vi "GetJSONData.vi"(0 "reference in":refnum<class "Graph.lvclass">, 2 "VI Reference":refnum<vi>, 5 "error in (no error)":errorcluster) -> (14 "reference out":refnum<class "Graph.lvclass">, 15 "JSON string":string, 19 "error out":errorcluster)   [LabVIEW 2014, in "Graph.lvclass"]
uses:
  Graph.lvclass
  <vilib>/Analysis/1siggen.llb/Ramp Pattern by Samples.vi
  <userlib>/_OpenG.lib/array/array.llb/Remove Duplicates from 1D Array (U32)__ogtk.vi
  <userlib>/_OpenG.lib/array/array.llb/Delete Elements from 1D Array (String)__ogtk.vi
  Object_class/Object.lvclass
  <vilib>/gmath/NI_Gmath.lvlib
  <vilib>/Analysis/NI_AALBase.lvlib
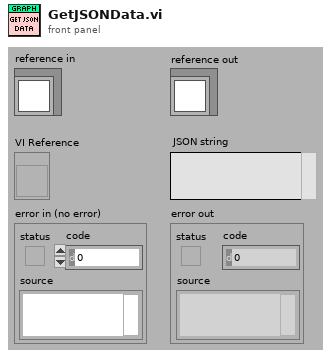
[diagram p1: front panel]
types:
  T1 = typedef "Object.lvclass/Attributes.ctl" = cluster{"UID":i32, "Type":string, "Coordinates":T2, "Reference":refnum<vi>}
  T2 = typedef "Object.lvclass/Coordinates.ctl" = cluster{"Left":i32, "Top":i32, "Height":u32, "Width":u32}
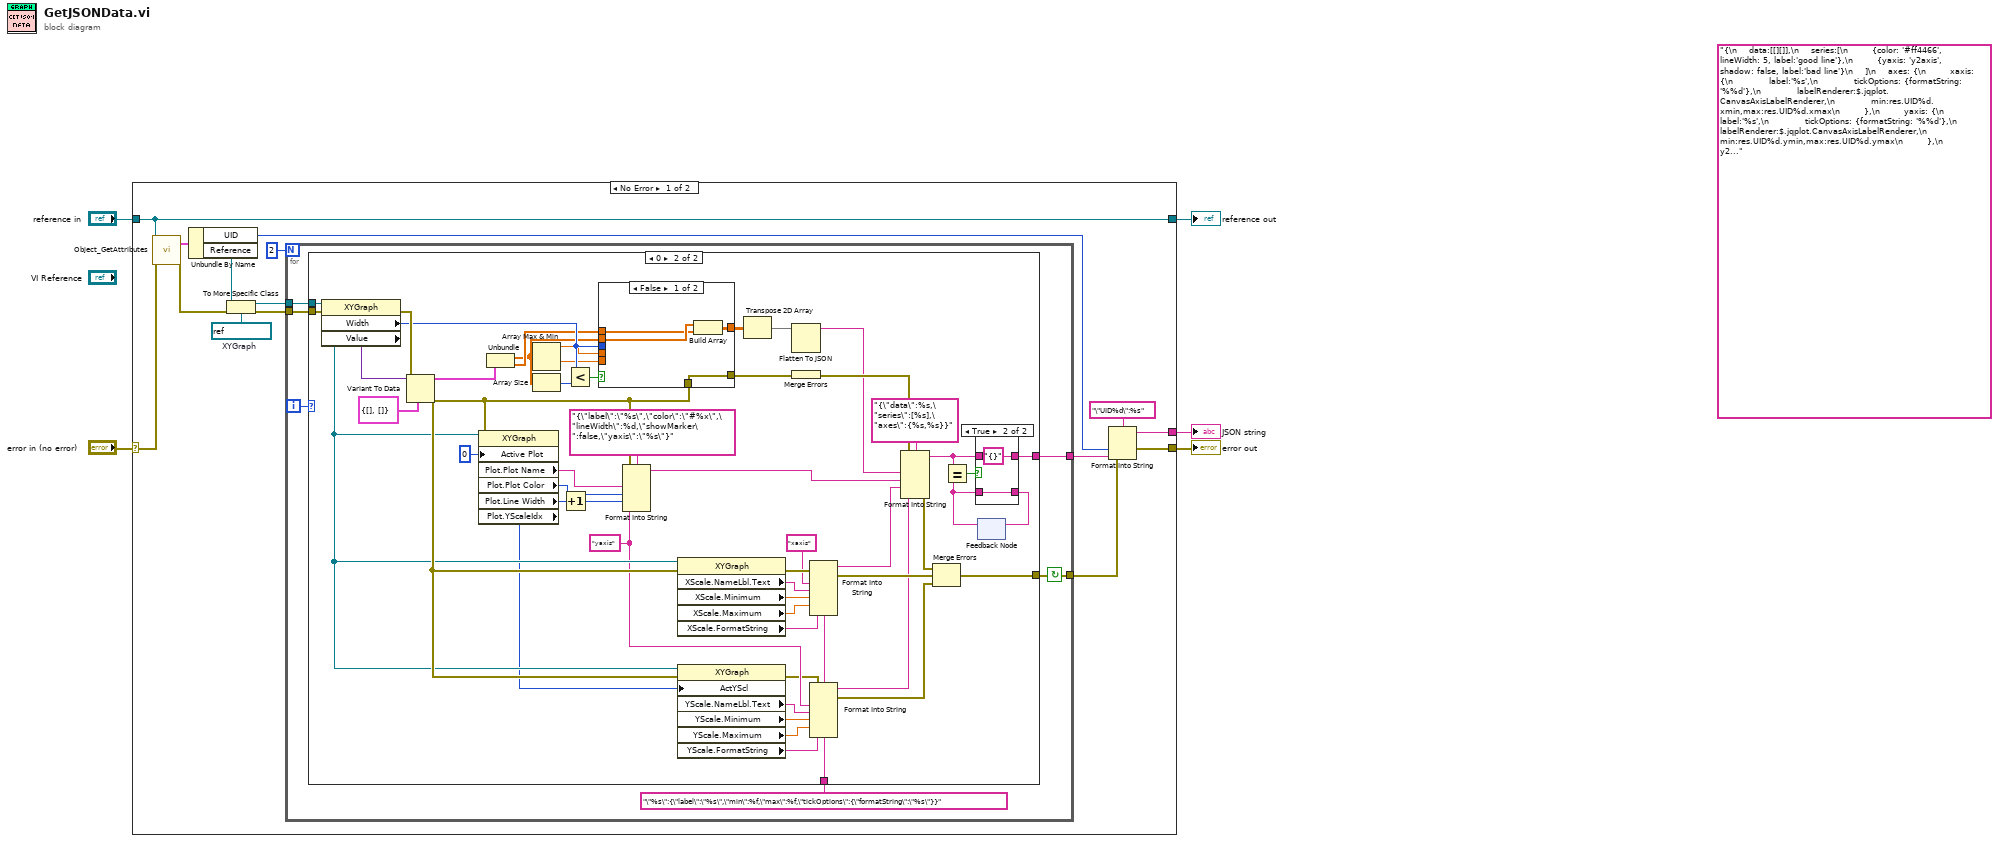
[diagram p0: block diagram]
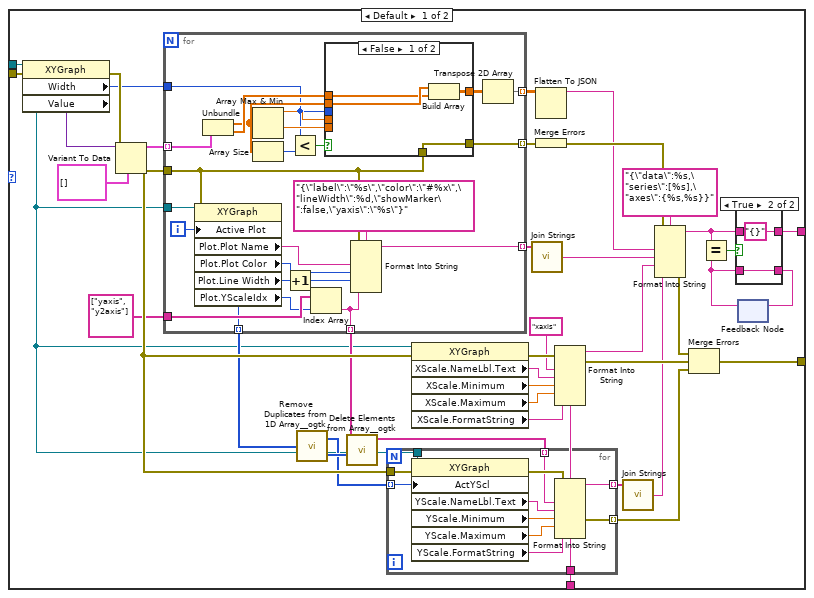
[diagram p2: hidden frame]
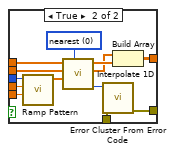
[diagram p4: hidden frame]
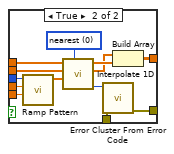
[diagram p5: hidden frame]
diagram:
  (unwired) "{\n    data:[[][]],\n    series:[\n        {color: '#ff4466', lineWidth: 5, label:'good line'},\n        {yaxis: 'y2axis', shadow: false, label:'bad line'}\n    ]\n    axes: {\n        xaxis: {\n            label:'%s',\n            tickOptions: {formatString: '%%d'},\n            labelRenderer:$.jqplot.CanvasAxisLabelRenderer,\n            min:res.UID%d.xmin,max:res.UID%d.xmax\n        },\n        yaxis: {\n            label:'%s',\n            tickOptions: {formatString: '%%d'},\n            labelRenderer:$.jqplot.CanvasAxisLabelRenderer,\n            min:res.UID%d.ymin,max:res.UID%d.ymax\n        },\n        y2axis: {\n            label:'%s',\n            tickOptions: {formatString: '%%d'},\n            labelRenderer:$.jqplot.CanvasAxisLabelRenderer\n        }\n      resetAxes:true\n    }\n}"
  n1 = case shown="No Error" "error in (no error)" {
    selector: "error in (no error)" -> [w18 w195]
    tunnel: [w19 w195] -> w4
    tunnel: [w11 w194] -> w2
    tunnel: "reference in" -> [w11 w194]
    tunnel: [w8 _] -> w1
    frame No Error {
      w12 = refnum<vi> refnum  # XYGraph
      n2 = call "Object_GetAttributes.vi"("reference in"=w11, "error in (no error)"=w18) -> ("Data"=w14:T1, "error out"=w16:errorcluster)  [unwired: 14 in, 2 out]
      n3 = Unbundle By Name(w14) -> ("UID"=w13:i32, "Reference"=w7:refnum<vi>)
      n4 = To More Specific Class(target class=w12, reference=w7, error in=w16) -> (specific class reference=w9:refnum<vi>, error out=w17:errorcluster)
      n5 = for {
        N: 2 -> [_]
        tunnel: [w25] -> w20
        tunnel: w17 -> [w26]
        tunnel: w9 -> [w23]
        tunnel: [w21] -> w6
        i -> [w24]
        stop <- w25 continue-if-true
        n6 = case shown="0" w24 {
          tunnel: w23 -> [w29 w147]
          tunnel: w26 -> [w60 w167]
          tunnel: [w59 w166] -> w25
          tunnel: "\"%s\":{\"label\":\"%s\",\"min\":%f,\"max\":%f,\"tickOptions\":{\"formatString\":\"%s\"}}" -> [w28 w146]
          tunnel: [w27 w145] -> w21
          frame Default {
            n7 = property class="XYGraph"(reference=w29, error in=w60) -> (error out=w66:errorcluster, "Width"=w34:u32, "Value"=w56:variant)  [unwired: 1 out]
            n8 = Variant To Data(error in=w66, type=cluster{dbl[], dbl[]}[] [], Variant=w56) -> (data=w54:cluster{dbl[], dbl[]}[], error out=w65:errorcluster)
            n9 = for {
              tunnel: [w102] -> w36 mode=indexing
              tunnel: w54 -> [w99] mode=indexing
              tunnel: w29 -> [w86]
              tunnel: [w104] -> w58 mode=indexing
              tunnel: w34 -> [w93]
              tunnel: w65 -> [w103]
              tunnel: string[] ["yaxis", "y2axis"] -> [w87]
              tunnel: [w85] -> w39 mode=indexing
              tunnel: [w84] -> w38 mode=indexing
              tunnel: [w83] -> w37 mode=indexing
              i -> [w88]
              n10 = property on="Property Node" class="XYGraph"(reference=w86, error in=w103, "Active Plot"=w88) -> ("Plot.Plot Name"=w90:string, "Plot.Plot Color"=w91:u32, "Plot.Line Width"=w92:u8, "Plot.YScaleIdx"=w85:u32)  [unwired: 2 out]
              n11 = Unbundle(w99) -> (w95:dbl[], w100:dbl[])
              n12 = Array Max & Min(array=w95) -> (max value=w98:dbl, min value=w97:dbl)  [unwired: 2 out]
              n13 = Array Size(array=w95) -> (size(s)=w94:i32)
              n14 = Increment(x=w92) -> (x+1=w82:u8)
              n15 = Less?(x=w93, y=w94) -> (x < y?=w96:bool)
              n16 = Index Array(array=w87, index=w85) -> (element=w84:string)
              n17 = case shown="False" w96 {
                tunnel: [w108 w121] -> w104
                tunnel: [w107 w119] -> w101
                tunnel: w100 -> [w105 w118]
                tunnel: w95 -> [w106 w112]
                tunnel: w98 -> [_ w111]
                tunnel: w97 -> [_ w110]
                tunnel: w93 -> [_ w109]
                tunnel: w103 -> [w108 w120]
                frame False {
                  n18 = Build Array(w106, w105) -> (w107:dbl[][])
                }
                frame True {
                  w113 = 0 items=["nearest", "linear", "spline", "cubic Hermite", "Lagrange"] ("method")
                  n19 = call-poly <vilib>:"Ramp Pattern.vi"("start"=w110, "end"=w111, "samples"=w109) -> ("Ramp Pattern"=w114:dbl[])  [unwired: 7 in, 1 out]
                  n20 = call <vilib>:"Interpolate 1D.vi"("method"=w113, "xi"=w114, "X"=w112, "Y"=w118) -> ("error"=w115:i32, "xi used"=w116:dbl[], "yi"=w117:dbl[])  [unwired: 5 in]
                  n21 = call <vilib>:"Error Cluster From Error Code.vi"("error in (no error)"=w120, "error code (0)"=w115) -> ("error out"=w121:errorcluster)  [unwired: 7 in]
                  n22 = Build Array(w116, w117) -> (w119:dbl[][])
                }
              }
              n23 = Format Into String(format string="{\"label\":\"%s\",\"color\":\"#%x\",\"lineWidth\":%d,\"showMarker\":false,\"yaxis\":\"%s\"}", error in=w103, w90, w91, w82, w84) -> (resulting string=w83:string)  [unwired: 1 in, 1 out]
              n24 = Transpose 2D Array(2D array=w101) -> (transposed array=w102:dbl[][])
            }
            n25 = call-poly <userlib>:"Remove Duplicates from 1D Array__ogtk.vi"("Input Array"=w39) -> ("Output Array"=w40:u32[], "indices of removed elements"=w51:i32[])
            n26 = call-poly <userlib>:"Delete Elements from Array__ogtk.vi"("indices"=w51, "array"=w38) -> ("array w/ subset deleted"=w52:string[])  [unwired: 8 in, 1 out]
            n27 = for {
              tunnel: w40 -> [w78] mode=indexing
              tunnel: w52 -> [w76] mode=indexing
              tunnel: [w72] -> w41 mode=indexing
              tunnel: w28 -> [w71]
              tunnel: w29 -> [w70]
              tunnel: w65 -> [w81]
              tunnel: [w79] -> w57 mode=indexing
              n28 = property on="Property Node" class="XYGraph"(reference=w70, error in=w81, "ActYScl"=w78) -> (error out=w80:errorcluster, "YScale.NameLbl.Text"=w77:string, "YScale.Minimum"=w75:dbl, "YScale.Maximum"=w74:dbl, "YScale.FormatString"=w73:string)  [unwired: 1 out]
              n29 = Format Into String(format string=w71, error in=w80, w76, w77, w75, w74, w73) -> (resulting string=w72:string, error out=w79:errorcluster)  [unwired: 1 in]
            }
            n30 = property on="Property Node" class="XYGraph"(reference=w29, error in=w65) -> (error out=w64:errorcluster, "XScale.NameLbl.Text"=w45:string, "XScale.Minimum"=w46:dbl, "XScale.Maximum"=w47:dbl, "XScale.FormatString"=w48:string)  [unwired: 1 out]
            n31 = call <vilib>:"Join Strings.vi"("Strings In"=w37) -> ("String"=w44:string)  [unwired: 2 in]
            n32 = Flatten To JSON(anything=w36) -> (JSON string=w35:string)  [unwired: 2 in, 1 out]
            n33 = Merge Errors(w58) -> (w63:errorcluster)
            n34 = Format Into String(format string=w28, error in=w64, "xaxis", w45, w46, w47, w48) -> (resulting string=w49:string, error out=w62:errorcluster)  [unwired: 1 in]
            n35 = call <vilib>:"Join Strings.vi"("Strings In"=w41) -> ("String"=w43:string)  [unwired: 2 in]
            n36 = Format Into String(format string="{\"data\":%s,\"series\":[%s],\"axes\":{%s,%s}}", error in=w63, w35, w44, w49, w43) -> (resulting string=w30:string, error out=w61:errorcluster)  [unwired: 1 in]
            n37 = Merge Errors(w61, w62, w57) -> (w59:errorcluster)
            n38 = feedback #1() -> (w31:string)  [unwired: 1 in]
            n39 = Equal?(x=w30, y=w31) -> (x = y?=w33:bool)
            n40 = case shown="True" w33 {
              tunnel: [w67 w69] -> w32
              tunnel: w31 -> [_ w69]
              tunnel: w30 -> [w67 _]
              tunnel: [w67 "{}"] -> w27
              frame False {
              }
              frame True {
              }
            }
            n41 = feedback-in #1(w32) -> ()
          }
          frame 0 {
            w129 = "yaxis"
            n42 = property class="XYGraph"(reference=w147, error in=w167) -> (error out=w173:errorcluster, "Width"=w152:u32, "Value"=w163:variant)  [unwired: 1 out]
            n43 = Variant To Data(error in=w173, type=cluster{dbl[], dbl[]} {[], []}, Variant=w163) -> (data=w162:cluster{dbl[], dbl[]}, error out=w172:errorcluster)
            n44 = property on="Property Node" class="XYGraph"(reference=w147, error in=w172, "Active Plot"=u32 0) -> ("Plot.Plot Name"=w134:string, "Plot.Plot Color"=w135:u32, "Plot.Line Width"=w136:u8, "Plot.YScaleIdx"=w128:u32)  [unwired: 2 out]
            n45 = Unbundle(w162) -> (w138:dbl[], w142:dbl[])
            n46 = Array Max & Min(array=w138) -> (max value=w141:dbl, min value=w140:dbl)  [unwired: 2 out]
            n47 = Array Size(array=w138) -> (size(s)=w137:i32)
            n48 = Increment(x=w136) -> (x+1=w132:u8)
            n49 = Less?(x=w152, y=w137) -> (x < y?=w139:bool)
            n50 = case shown="False" w139 {
              tunnel: [w177 w190] -> w165
              tunnel: [w176 w188] -> w143
              tunnel: w142 -> [w174 w187]
              tunnel: w138 -> [w175 w181]
              tunnel: w141 -> [_ w180]
              tunnel: w140 -> [_ w179]
              tunnel: w152 -> [_ w178]
              tunnel: w172 -> [w177 w189]
              frame False {
                n51 = Build Array(w175, w174) -> (w176:dbl[][])
              }
              frame True {
                w182 = 0 items=["nearest", "linear", "spline", "cubic Hermite", "Lagrange"] ("method")
                n52 = call-poly <vilib>:"Ramp Pattern.vi"("start"=w179, "end"=w180, "samples"=w178) -> ("Ramp Pattern"=w183:dbl[])  [unwired: 7 in, 1 out]
                n53 = call <vilib>:"Interpolate 1D.vi"("method"=w182, "xi"=w183, "X"=w181, "Y"=w187) -> ("error"=w184:i32, "xi used"=w185:dbl[], "yi"=w186:dbl[])  [unwired: 5 in]
                n54 = call <vilib>:"Error Cluster From Error Code.vi"("error in (no error)"=w189, "error code (0)"=w184) -> ("error out"=w190:errorcluster)  [unwired: 7 in]
                n55 = Build Array(w185, w186) -> (w188:dbl[][])
              }
            }
            n56 = Format Into String(format string="{\"label\":\"%s\",\"color\":\"#%x\",\"lineWidth\":%d,\"showMarker\":false,\"yaxis\":\"%s\"}", error in=w172, w134, w135, w132, w129) -> (resulting string=w130:string)  [unwired: 1 in, 1 out]
            n57 = property on="Property Node" class="XYGraph"(reference=w147, error in=w172) -> (error out=w171:errorcluster, "XScale.NameLbl.Text"=w156:string, "XScale.Minimum"=w157:dbl, "XScale.Maximum"=w158:dbl, "XScale.FormatString"=w159:string)  [unwired: 1 out]
            n58 = property on="Property Node" class="XYGraph"(reference=w147, error in=w172, "ActYScl"=w128) -> (error out=w127:errorcluster, "YScale.NameLbl.Text"=w126:string, "YScale.Minimum"=w125:dbl, "YScale.Maximum"=w124:dbl, "YScale.FormatString"=w123:string)  [unwired: 1 out]
            n59 = Transpose 2D Array(2D array=w143) -> (transposed array=w154:dbl[][])
            n60 = Flatten To JSON(anything=w154) -> (JSON string=w153:string)  [unwired: 2 in, 1 out]
            n61 = Merge Errors(w165) -> (w170:errorcluster)
            n62 = Format Into String(format string=w146, error in=w171, "xaxis", w156, w157, w158, w159) -> (resulting string=w160:string, error out=w169:errorcluster)  [unwired: 1 in]
            n63 = Format Into String(format string=w146, error in=w127, w129, w126, w125, w124, w123) -> (resulting string=w122:string, error out=w164:errorcluster)  [unwired: 1 in]
            n64 = Format Into String(format string="{\"data\":%s,\"series\":[%s],\"axes\":{%s,%s}}", error in=w170, w153, w130, w160, w122) -> (resulting string=w148:string, error out=w168:errorcluster)  [unwired: 1 in]
            n65 = Merge Errors(w168, w169, w164) -> (w166:errorcluster)
            n66 = feedback #2() -> (w149:string)  [unwired: 1 in]
            n67 = Equal?(x=w148, y=w149) -> (x = y?=w151:bool)
            n68 = case shown="True" w151 {
              tunnel: [w191 w193] -> w150
              tunnel: w149 -> [_ w193]
              tunnel: w148 -> [w191 _]
              tunnel: [w191 "{}"] -> w145
              frame False {
              }
              frame True {
              }
            }
            n69 = feedback-in #2(w150) -> ()
          }
        }
      }
      n70 = Format Into String(format string="\"UID%d\":%s", error in=w20, w13, w6) -> (resulting string=w8:string, error out=w19:errorcluster)  [unwired: 1 in]
    }
    frame Error {
    }
  }
  "error out" <- w4
  "reference out" <- w2
  "JSON string" <- w1
